vi "createSetForceFrame.vi"(0 "SAAILC in":refnum<class "SAAILC.lvclass">, 5 "WaitForTrigger":bool, 7 "TriggerIRQ":bool, 9 "SlewFlag":bool, 11 "error in (no error)":errorcluster) -> (4 "SAAILC out":refnum<class "SAAILC.lvclass">, 6 "TxFrame":T1 {"Data" format="%02x"}, 15 "error out":errorcluster)   [LabVIEW 2016, in "RTFAILC.lvlib" / "SAAILC.lvclass"]
uses:
  SAAILC.lvclass
  D:/Code/Common_RT_ILC/ILC/ILC.lvclass
  D:/Code/Common_RT_FAILC/FAILC/FAILC.lvclass
  Common_RT_Modbus/DataTypes/TxFrame.ctl
  Common_RT_Modbus/DynamicFrameBuilder/DynamicFrameBuilder.lvclass
  FAILC/FAILC.lvclass/FAILC.ctl
  Common_RT_ILC/ILC/ILC.lvclass/ILC.ctl
  Common_RT_ILC/ILC/ILC.lvclass
  FAILC/FAILC.lvclass
  Common_RT_Modbus/RTModbus.lvlib
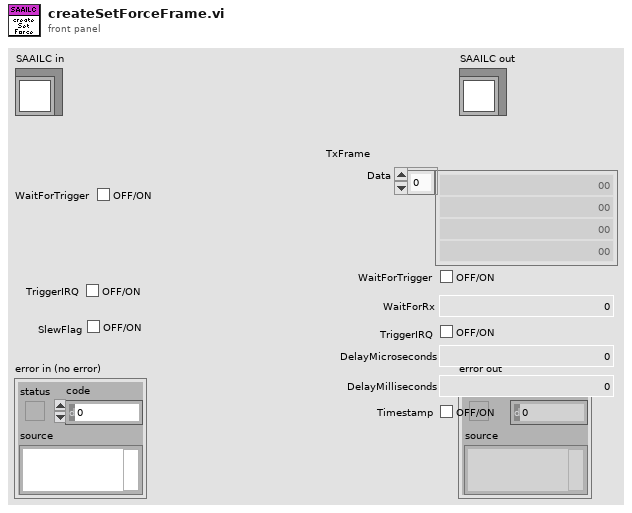
[diagram p1: front panel]
types:
  T1 = typedef "RTModbus.lvlib/TxFrame.ctl" = cluster{"Data":u8[], "WaitForTrigger":bool, "WaitForRx":u16, "TriggerIRQ":bool, "DelayMicroseconds":u16, "DelayMilliseconds":u16, "Timestamp":bool}
  T2 = typedef "RTILC.lvlib/ILCData.ctl" = cluster{"Constants":T3, "Command":T4, "Telemetry":T6, "Responses":T7, "Timings":T9}
  T3 = typedef "RTILC.lvlib/ILCConstants.ctl" = cluster{"Subnet":u8, "Address":u8}
  T4 = typedef "RTILC.lvlib/ILCCommand.ctl" = cluster{"ILCMode":u16, "TemporaryAddress":u8, "ADCScanRate":T5, "ADCChannel":u8, "ADCOffset":sgl, "ADCSensitivity":sgl}
  T5 = typedef "RTILC.lvlib/ILCScanRates.ctl" = u8
  T6 = typedef "RTILC.lvlib/ILCTelemetry.ctl" = cluster{"UniqueID":u64, "FirmwareType":u8, "NetworkNodeType":u8, "ILCOption":u8, "NetworkNodeOption":u8, "MajorRevision":u8, "MinorRevision":u8, "FirmwareName":string, "ILCMode":u16, "MajorFault":bool, "MinorFault":bool, "FaultOverride":bool, "UniqueIDCRCMismatch":bool, "AppTypeNodeTypeMismatch":bool, "AppMissing":bool, "AppCRCMismatch":bool, "TEDSNotFound":bool, "TEDS1Mismatch":bool, "TEDS2Mismatch":bool, "WatchdogResetDetected":bool, "BrownoutDetected":bool, "EventTrapResetDetected":bool, "TemporaryAddress":u8, "ADCScanRate":T5, "DAC1":u16, "DAC2":u16, "DAC3":u16, "DAC4":u16, "MainADCCalibrationK":sgl[], "MainSensorOffset":sgl[], "MainSensorSensitivity":sgl[], "BackupADCCalibrationK":sgl[], "BackupSensorOffset":sgl[], "BackupSensorSensitivity":sgl[]}
  T7 = typedef "RTILC.lvlib/ILCResponses.ctl" = cluster{"ReportServerID":T8, "ReportServerStatus":T8, "ILCMode":T8, "SetTemporaryAddress":T8, "Reset":T8, "ADCScanRate":T8, "ADCOffsetSensitivity":T8, "ReadDAC":T8, "ReadCalibration":T8}
  T8 = typedef "RTModbus.lvlib/ExceptionCodes.ctl" = u16
  T9 = typedef "RTILC.lvlib/ILCTimings.ctl" = cluster{"ADCOffsetSensitivity":u32, "ADCScanRate":u32, "ILCMode":u32, "ReadCalibration":u32, "ReportServerID":u32, "ReportServerStatus":u32, "Reset":u32, "SetTemporaryAddress":u32}
  T10 = typedef "RTFAILC.lvlib/FAData.ctl" = cluster{"Constants":T11, "Command":T12, "Telemetry":T13, "Responses":T14, "Timings":T15}
  T11 = typedef "RTFAILC.lvlib/FAConstants.ctl" = cluster{"ID":i16}
  T12 = typedef "RTFAILC.lvlib/FACommand.ctl" = cluster{"AxialSetPoint":i32, "LateralSetPoint":i32, "AxialBoosterValveGain":sgl, "LateralBoosterValveGain":sgl}
  T13 = typedef "RTFAILC.lvlib/FATelemetry.ctl" = cluster{"ILCFault":bool, "BroadcastCounter":u8, "AxialLoadCellForce":sgl, "LateralLoadCellForce":sgl, "AxialBoosterValveGain":sgl, "LateralBoosterValveGain":sgl}
  T14 = typedef "RTFAILC.lvlib/FAResponses.ctl" = cluster{"BoosterValveGain":T8, "ReadBoosterValveGain":T8, "SetForce":T8, "ForceAndStatus":T8}
  T15 = typedef "RTFAILC.lvlib/FATimings.ctl" = cluster{"BroadcastSetForce":u32, "BoosterValveGain":u32, "FreezeSensorValues":u32, "ForceAndStatus":u32, "ReadBoosterValveGain":u32, "SetForce":u32}
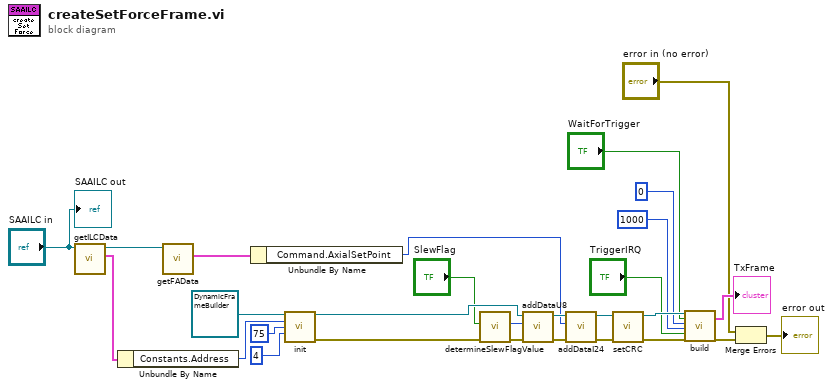
[diagram p0: block diagram]
diagram:
  n1 = call "getILCData.vi"("ILC in"="SAAILC in") -> ("ILCData"=w27:T2, "ILC out"=w28:refnum<class "SAAILC.lvclass">)  [unwired: 9 in]
  n2 = Unbundle By Name(w27) -> ("Constants.Address"=w24:u8)
  n3 = call "getFAData.vi"("FAILC in"=w28) -> ("FAData"=w26:T10)  [unwired: 9 in, 1 out]
  n4 = Unbundle By Name(w26) -> ("Command.AxialSetPoint"=w6:i32)
  n5 = call "init.vi"("DynamicFrameBuilder in"=refnum<class "DynamicFrameBuilder.lvclass"> refnum ("RTModbus.lvlib:DynamicFrameBuilder.lvclass"), "Address"=w24, "Function"=u8 75, "DataSize"=4) -> ("DynamicFrameBuilder out"=w21:refnum<class "DynamicFrameBuilder.lvclass">, "error out"=w2:errorcluster)  [unwired: 10 in]
  n6 = call "determineSlewFlagValue.vi"("error in (no error)"=w2, "SlewFlag"="SlewFlag") -> ("error out"=w1:errorcluster, "FlagValue"=w3:u8)  [unwired: 7 in, 1 out]
  n7 = call "addDataU8.vi"("error in (no error)"=w1, "Data"=w3, "DynamicFrameBuilder in"=w21) -> ("error out"=w19:errorcluster, "DynamicFrameBuilder out"=w20:refnum<class "DynamicFrameBuilder.lvclass">)  [unwired: 7 in]
  n8 = call "addDataI24.vi"("error in (no error)"=w19, "Data"=w6, "DynamicFrameBuilder in"=w20) -> ("error out"=w18:errorcluster, "DynamicFrameBuilder out"=w17:refnum<class "DynamicFrameBuilder.lvclass">)  [unwired: 7 in]
  n9 = call "setCRC.vi"("error in (no error)"=w18, "DynamicFrameBuilder in"=w17) -> ("error out"=w12:errorcluster, "DynamicFrameBuilder out"=w16:refnum<class "DynamicFrameBuilder.lvclass">)  [unwired: 8 in]
  n10 = call "build.vi"("DynamicFrameBuilder in"=w16, "WaitForTrigger"="WaitForTrigger", "Latency"=u32 0, "WaitForRxTimeout"=u16 1000, "TriggerIRQ"="TriggerIRQ", "error in (no error)"=w12) -> ("TxFrame"=→"TxFrame":T1, "error out"=w10:errorcluster)  [unwired: 11 in, 1 out]
  n11 = Merge Errors("error in (no error)", w10) -> (→"error out":errorcluster)
  "SAAILC out" <- "SAAILC in"
